vi "front pannel close.vi"(8 "错误输入（无错误）":errorcluster) -> (0 "错误输出":errorcluster)   [LabVIEW 2020]
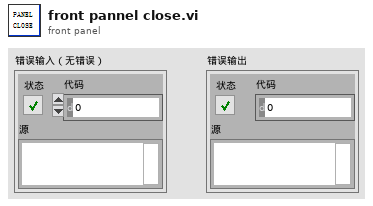
[diagram p1: front panel]
types:
  T1 = enum32{"invalid app kind", "Development System", "Run Time System", "Student Edition", "Embedded LabVIEW", "Evaluation", "Custom"}
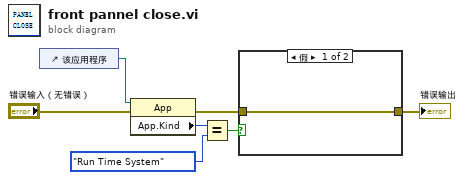
[diagram p0: block diagram]
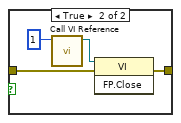
[diagram p2: hidden frame]
diagram:
  n1 = control-ref of="该应用程序"() -> (w5:refnum<vi>)
  n2 = property class="App"(reference=w5, error in="错误输入（无错误）") -> (error out=w6:errorcluster, "App.Kind"=w1:T1)  [unwired: 1 out]
  n3 = Equal?(x=w1, y=T1."Run Time System" ("x")) -> (x = y?=w7:bool)
  n4 = case shown="假" w7 {
    tunnel: w6 -> [w8 w12]
    tunnel: [w8 w9] -> w4
    frame False {
    }
    frame True {
      n5 = call "Call VI Reference.vi"("last level"=1 ("last level reference")) -> ("vi reference out"=w10:refnum<vi>)  [unwired: 9 in, 1 out]
      n6 = invoke class="VI" method="FP.Close"(reference=w10, error in=w12) -> (error out=w9:errorcluster)  [unwired: 1 in, 2 out]
    }
  }
  "错误输出" <- w4
